vi "about read folder notes to js.vi"(8 "error in (no error)":errorcluster, 11 "Modules Path (empty)":path) -> (0 "error out":errorcluster, 3 "Module Notes objects":string)   [LabVIEW 2011]
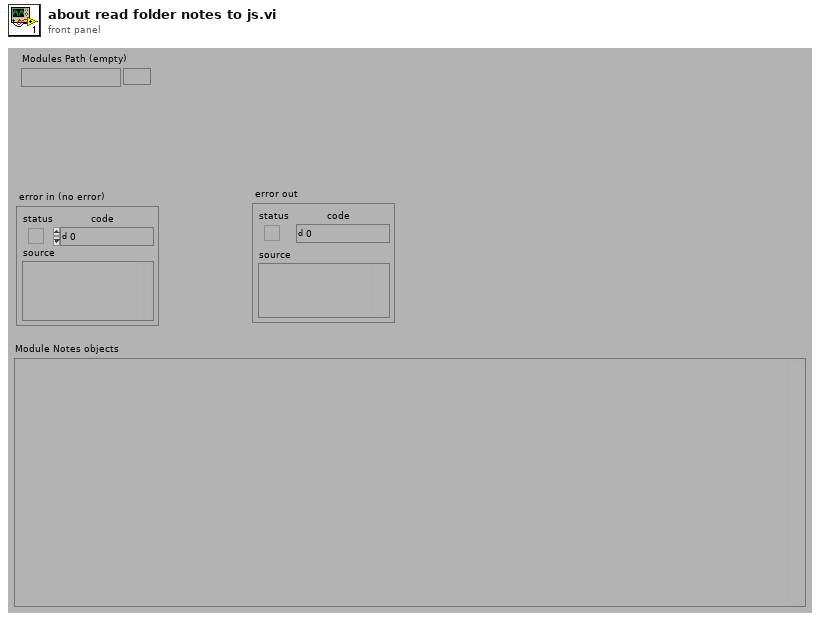
[diagram p1: front panel]
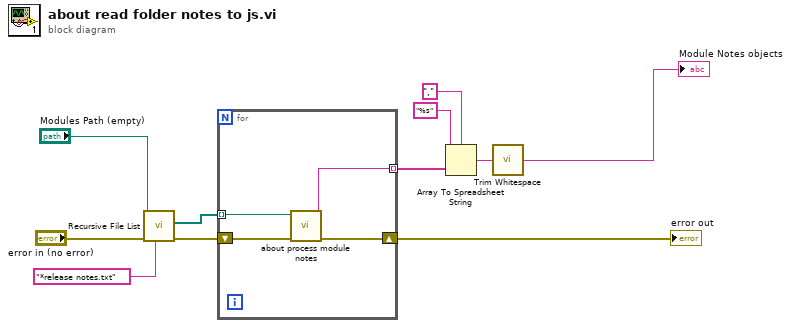
[diagram p0: block diagram]
diagram:
  n1 = call <vilib>:"Recursive File List.vi"("pattern"="*release notes.txt", "error in (no error)"="error in (no error)", "Folder Path"="Modules Path (empty)") -> ("error out"=w2:errorcluster, "All Files in Dir"=w1:path[])  [unwired: 1 in, 6 out]
  n2 = for {
    shift-right: [w14] -> w6
    shift-left: w2 -> [w15]
    tunnel: [w13] -> w11 mode=indexing
    tunnel: w1 -> [w12] mode=indexing
    n3 = call "about process module notes.vi"("error in (no error)"=w15, "Notes Path (empty)"=w12) -> ("error out"=w14:errorcluster, "release notes obj"=w13:string)  [unwired: 8 out]
  }
  "error out" <- w6
  n4 = Array To Spreadsheet String(delimiter (Tab)=",", array=w11, 3:"%s") -> (spreadsheet string=w8:string)
  n5 = call <vilib>:"Trim Whitespace.vi"("string"=w8) -> ("trimmed string"=→"Module Notes objects":string)  [unwired: 1 in]
